vi "Kalman.vi"(0 "x":dbl, 1 "y":dbl, 2 "theta":dbl, 3 "GPS X":dbl format="%#_13g", 4 "GPS Y":dbl format="%#_13g", 5 "GPS theta":dbl format="%#_13g", 7 "ds":dbl, 9 "phi":dbl, 11 "delta":dbl) -> (14 "new x":dbl, 15 "new y":dbl, 16 "new theta":dbl)   [LabVIEW 2016]
uses:
  <vilib>/Analysis/7linalg.llb/Real Transpose Matrix.vi
  <vilib>/Analysis/baseanly.llb/Real A x B.vi
  <vilib>/Analysis/Matrix/Numeric/Add/Add - RM,RM.vi
  <vilib>/Analysis/baseanly.llb/Real Inverse Matrix.vi
  <vilib>/Analysis/Matrix/Numeric/Subtract/Subtract - RM,RM.vi
  <vilib>/Analysis/NI_AALBase.lvlib
  <vilib>/Analysis/NI_AALPro.lvlib
  <vilib>/Analysis/Matrix/NI_Matrix.lvlib
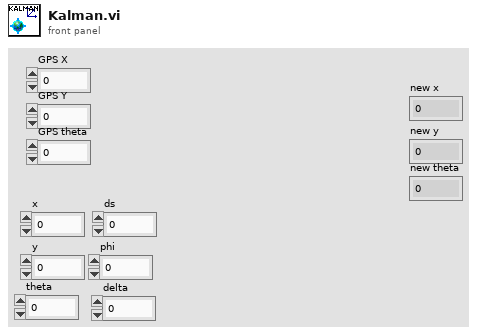
[diagram p1: front panel]
types:
  T1 = typedef "NI_Matrix.lvlib/RealMatrix.ctl" = dbl[][]
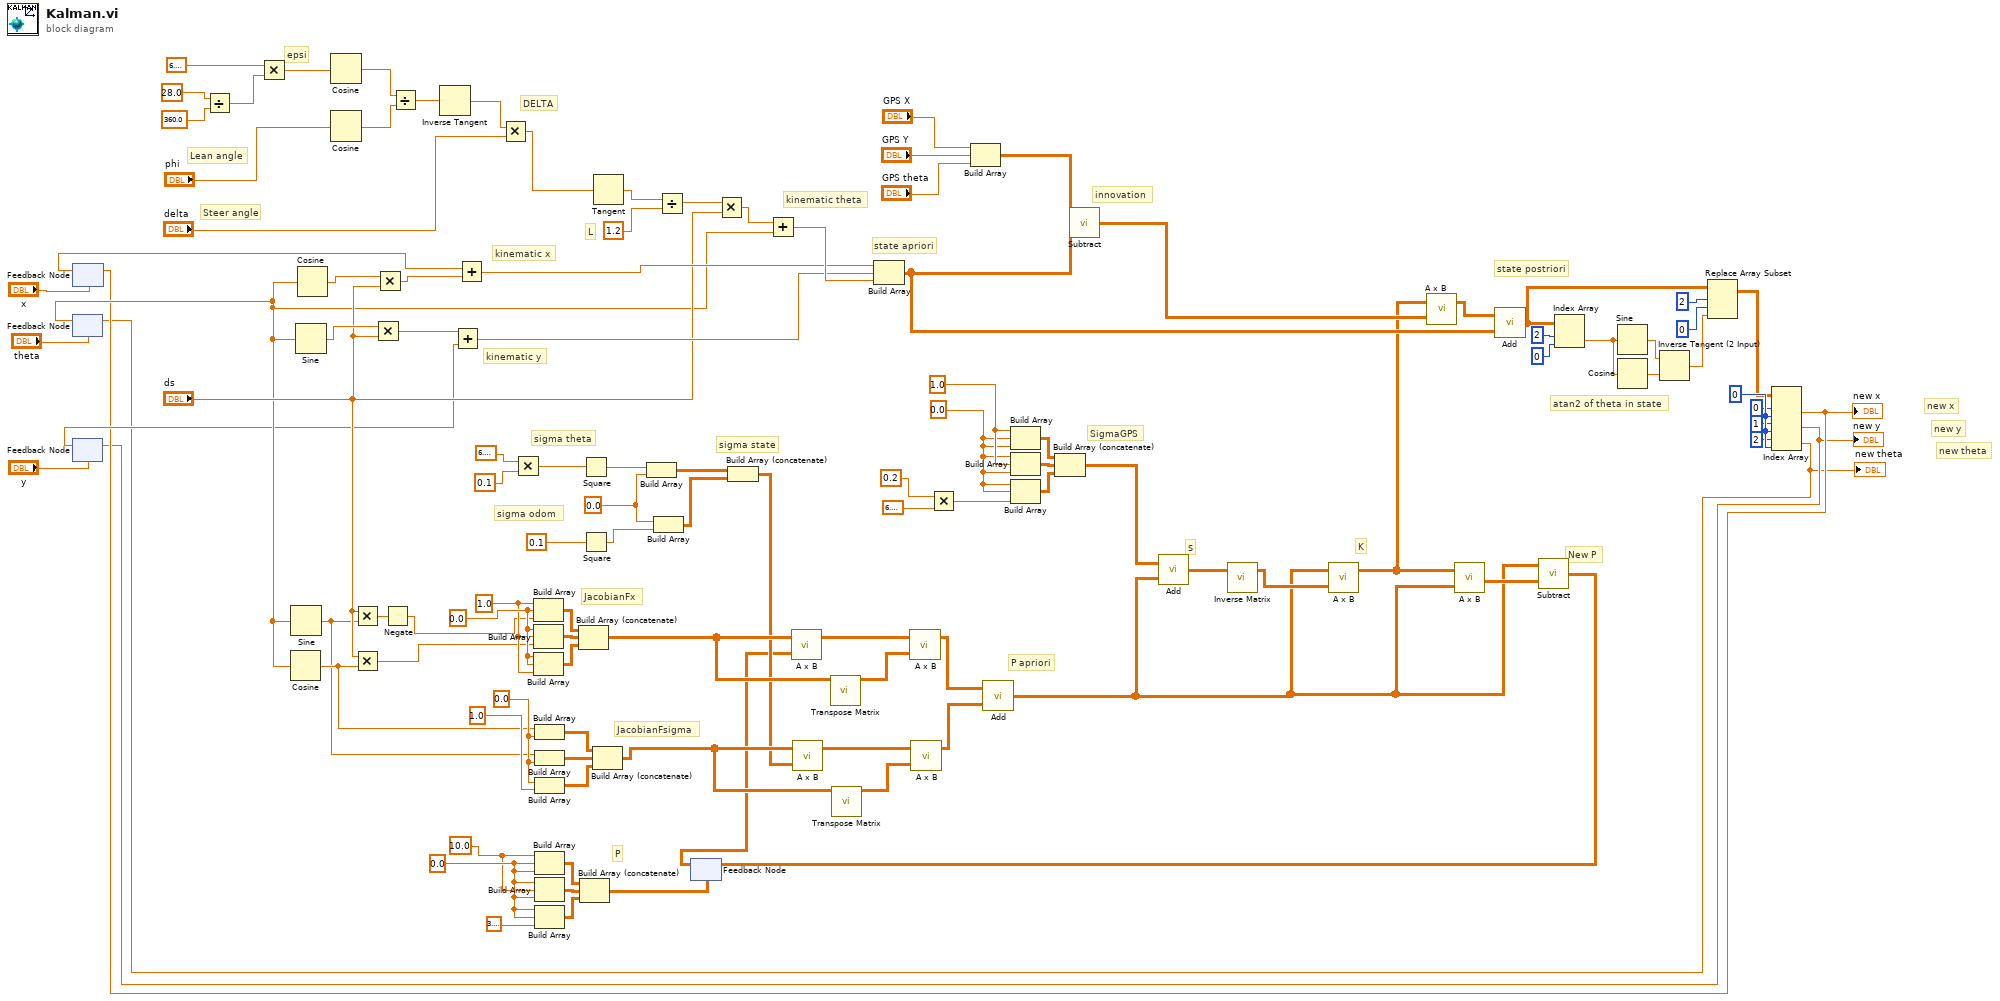
[diagram p0: block diagram]
diagram:
  w14 = 0 ("disabled index (col)")
  w42 = 0.0
  w43 = 1.0
  w59 = 0.0
  w57 = 10.0
  w69 = 0.0
  w75 = 0.0
  w74 = 1.0
  w80 = 0.0
  # "Lean angle"
  # "Steer angle"
  # "new theta"
  # "new y"
  # "new x"
  # "New P"
  # "atan2 of theta in state"
  # "state postriori"
  # "K"
  # "S"
  # "innovation"
  # "SigmaGPS"
  # "P apriori"
  # "P"
  # "JacobianFsigma"
  # "JacobianFx"
  # "sigma state"
  # "sigma odom"
  # "sigma theta"
  # "state apriori"
  # "kinematic theta"
  # "kinematic y"
  # "kinematic x"
  # "DELTA"
  # "L"
  # "epsi"
  n1 = feedback #1("theta") -> (w9:dbl)
  n2 = feedback #2("y") -> (w6:dbl)
  n3 = feedback #3("x") -> (w7:dbl)
  n4 = Divide(x=28.0, y=360.0) -> (x/y=w108:dbl)
  n5 = Multiply(x=6.283185307179586, y=w108) -> (x*y=w106:dbl)
  n6 = Cosine(x=w9) -> (cos(x)=w67:dbl)
  n7 = Sine(x=w9) -> (sin(x)=w66:dbl)
  n8 = Sine(x=w9) -> (sin(x)=w98:dbl)
  n9 = Cosine(x=w9) -> (cos(x)=w99:dbl)
  n10 = Cosine(x=w106) -> (cos(x)=w104:dbl)
  n11 = Cosine(x="phi") -> (cos(x)=w103:dbl)
  n12 = Multiply(x="ds", y=w66) -> (x*y=w73:dbl)
  n13 = Multiply(x="ds", y=w67) -> (x*y=w72:dbl)
  n14 = Multiply(x=w98, y="ds") -> (x*y=w97:dbl)
  n15 = Multiply(x=w99, y="ds") -> (x*y=w96:dbl)
  n16 = Negate(x=w73) -> (-x=w71:dbl)
  n17 = Divide(x=w104, y=w103) -> (x/y=w102:dbl)
  n18 = Inverse Tangent(1:w102) -> (0:w101:dbl)
  n19 = Add(x=w97, y=w6) -> (x+y=w89:dbl)
  n20 = Add(x=w7, y=w96) -> (x+y=w88:dbl)
  n21 = Multiply(x=w101, y="delta") -> (x*y=w95:dbl)
  n22 = Multiply(x=6.283185307179586, y=0.1) -> (x*y=w85:dbl)
  n23 = Build Array(w74, w75, w71) -> (w78:T1)
  n24 = Build Array(w75, w74, w72) -> (w77:T1)
  n25 = Build Array(w75, w75, w74) -> (w76:T1)
  n26 = Build Array(w67, w69) -> (w65:T1)
  n27 = Build Array(w66, w69) -> (w64:T1)
  n28 = Build Array(w69, 1.0) -> (w63:T1)
  n29 = Build Array(w57, w59, w59) -> (w62:T1)
  n30 = Build Array(w59, w57, w59) -> (w61:T1)
  n31 = Build Array(w59, w59, 3.141592653589793) -> (w60:T1)
  n32 = Build Array (concatenate)(w78, w77, w76) -> (w55:T1)
  n33 = Build Array (concatenate)(w62, w61, w60) -> (w17:T1)
  n34 = Square(x=w85) -> (x^2=w83:dbl)
  n35 = Square(x=0.1) -> (x^2=w81:dbl)
  n36 = Build Array (concatenate)(w65, w64, w63) -> (w51:T1)
  n37 = Tangent(1:w95) -> (0:w94:dbl)
  n38 = Build Array(w83, w80) -> (w82:T1)
  n39 = Build Array(w80, w81) -> (w79:T1)
  n40 = Divide(x=w94, y=1.2) -> (x/y=w92:dbl)
  n41 = feedback #4(w17) -> (w16:T1)
  n42 = Multiply(x=w92, y="ds") -> (x*y=w91:dbl)
  n43 = Build Array (concatenate)(w82, w79) -> (w50:T1)
  n44 = Add(x=w91, y=w9) -> (x+y=w90:dbl)
  n45 = call-poly <vilib>:"A x B.vi"("B"=w16, "A"=w55) -> ("A x B"=w56:T1)  [unwired: 1 out]
  n46 = call-poly <vilib>:"A x B.vi"("B"=w50, "A"=w51) -> ("A x B"=w52:T1)  [unwired: 1 out]
  n47 = call-poly <vilib>:"Transpose Matrix.vi"("Input Matrix"=w55) -> ("Matrix Transpose"=w54:T1)  [unwired: 9 in, 1 out]
  n48 = call-poly <vilib>:"Transpose Matrix.vi"("Input Matrix"=w51) -> ("Matrix Transpose"=w53:T1)  [unwired: 9 in, 1 out]
  n49 = Build Array(w88, w89, w90) -> (w31:T1)
  n50 = call-poly <vilib>:"A x B.vi"("B"=w54, "A"=w56) -> ("A x B"=w49:T1)  [unwired: 1 out]
  n51 = call-poly <vilib>:"A x B.vi"("B"=w53, "A"=w52) -> ("A x B"=w48:T1)  [unwired: 1 out]
  n52 = Multiply(x=0.2, y=6.283185307179586) -> (x*y=w40:dbl)
  n53 = Build Array("GPS X", "GPS Y", "GPS theta") -> (w36:T1)
  n54 = call-poly <vilib>:"Add.vi"("Real Matrix B"=w48, "Real Matrix A"=w49) -> ("A + B"=w18:T1)
  n55 = Build Array(w43, w42, w42) -> (w46:T1)
  n56 = Build Array(w42, w43, w42) -> (w45:T1)
  n57 = Build Array(w42, w42, w40) -> (w44:T1)
  n58 = Build Array (concatenate)(w46, w45, w44) -> (w35:T1)
  n59 = call-poly <vilib>:"Subtract.vi"("Real Matrix B"=w31, "Real Matrix A"=w36) -> ("A - B"=w32:T1)
  n60 = call-poly <vilib>:"Add.vi"("Real Matrix B"=w18, "Real Matrix A"=w35) -> ("A + B"=w34:T1)
  n61 = call-poly <vilib>:"Inverse Matrix.vi"("Input Matrix"=w34) -> ("Inverse Matrix"=w33:T1)  [unwired: 1 in, 1 out]
  n62 = call-poly <vilib>:"A x B.vi"("B"=w33, "A"=w18) -> ("A x B"=w20:T1)  [unwired: 1 out]
  n63 = call-poly <vilib>:"A x B.vi"("B"=w32, "A"=w20) -> ("A x B"=w30:T1)  [unwired: 1 out]
  n64 = call-poly <vilib>:"A x B.vi"("B"=w18, "A"=w20) -> ("A x B"=w19:T1)  [unwired: 1 out]
  n65 = call-poly <vilib>:"Add.vi"("Real Matrix B"=w31, "Real Matrix A"=w30) -> ("A + B"=w24:T1)
  n66 = call-poly <vilib>:"Subtract.vi"("Real Matrix B"=w19, "Real Matrix A"=w18) -> ("A - B"=w15:T1)
  n67 = feedback-in #4(w15) -> ()
  n68 = Index Array(array=w24, index (row)=2, index (col)=0) -> (element=w27:dbl)
  n69 = Sine(x=w27) -> (sin(x)=w26:dbl)
  n70 = Cosine(x=w27) -> (cos(x)=w25:dbl)
  n71 = Inverse Tangent (2 Input)(1:w25, 2:w26) -> (0:w23:dbl)
  n72 = Replace Array Subset(array=w24, new element=w23, index (row)=2 ("disabled index (row)"), index (col)=0 ("disabled index (col)")) -> (w3:T1)
  n73 = Index Array(array=w3, index (row) #1=0 ("index (row)"), index (col) #1=w14, index (row) #2=1 ("index (row)"), index (col) #2=w14, index (row) #3=2 ("index (row)"), index (col) #3=w14) -> (element #1=w4:dbl, element #2=w2:dbl, element #3=w1:dbl)
  "new x" <- w4
  "new y" <- w2
  "new theta" <- w1
  n74 = feedback-in #1(w1) -> ()
  n75 = feedback-in #2(w2) -> ()
  n76 = feedback-in #3(w4) -> ()
